vi "LVCAM Nest Destroyed.vi"(9 "Nest Error":errorcluster, 10 "Nest Actor":refnum<class "Actor.lvclass">, 11 "Process in":refnum<class "ABD.lvclass">) -> (0 "error out":errorcluster, 3 "Process out":refnum<class "ABD.lvclass">)   [LabVIEW 2021, in "ABD.lvlib" / "ABD.lvclass"]
uses:
  ABD.lvclass
  LVCAM/LVCAM/Actor/Actor.lvclass
  ABD.lvclass/ABD.ctl
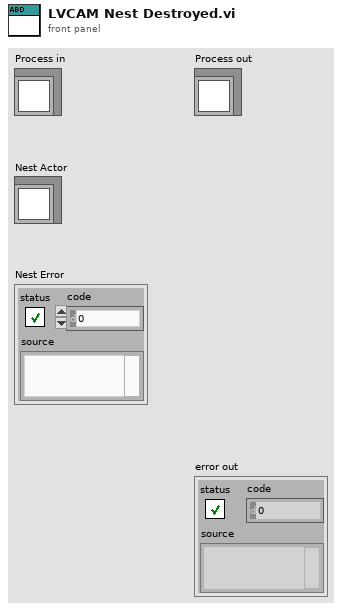
[diagram p1: front panel]
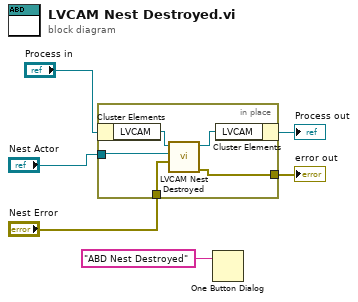
[diagram p0: block diagram]
diagram:
  n1 = in-place {
    in-place-border: "Nest Actor" -> [w9]
    in-place-border: [w8] -> w3
    in-place-border: "Nest Error" -> [w7]
    n2 = in-place-cluster #1("Process in") -> ("LVCAM"=w11:refnum<class "Actor.lvclass">)
    n3 = call-dynamic "LVCAM Nest Destroyed.vi"("Nest Error"=w7, "Nest Actor"=w9, "LVCAM Nest Destroyed in"=w11) -> ("error out"=w8:errorcluster, "LVCAM Nest Destroyed out"=w10:refnum<class "Actor.lvclass">)  [unwired: 7 in]
    n4 = in-place-cluster #1("LVCAM"=w10) -> (→"Process out":refnum<class "ABD.lvclass">)
  }
  "error out" <- w3
  n5 = One Button Dialog(message="ABD Nest Destroyed") -> ()  [unwired: 1 in, 1 out]
